vi "uPolicy_TopicIsRelevant.vi"(8 "error in (no error)":errorcluster, 10 "Observed Topic (Lower Case)":string, 11 "SelectTopics in":refnum<class "SelectTopics.lvclass">) -> (0 "error out":errorcluster, 2 "Relevant?":bool, 3 "SelectTopics out":refnum<class "SelectTopics.lvclass">)   [LabVIEW 2021, in "uFramework_pack_uPolicy.lvlib" / "SelectTopics.lvclass"]
uses:
  SelectTopics.lvclass
  SelectTopics.lvclass/SelectTopics.ctl
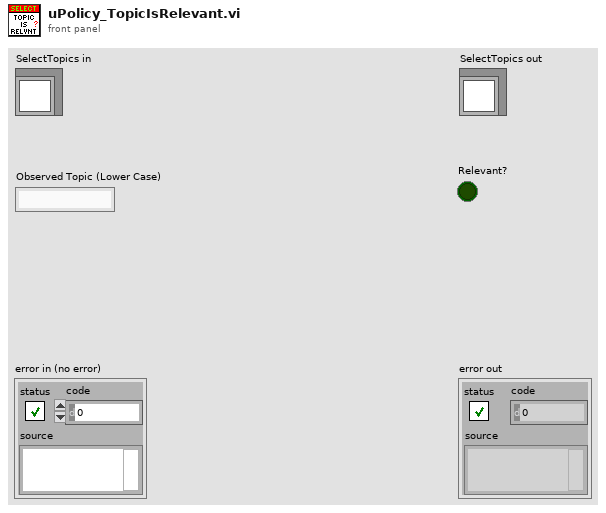
[diagram p1: front panel]
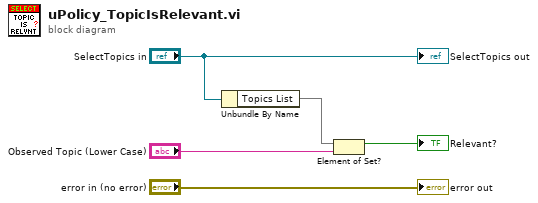
[diagram p0: block diagram]
diagram:
  n1 = Unbundle By Name("SelectTopics in") -> ("Topics List"=w3:set{string})
  n2 = Element of Set?(10:"Observed Topic (Lower Case)", 11:w3) -> (3:→"Relevant?":bool)
  "error out" <- "error in (no error)"
  "SelectTopics out" <- "SelectTopics in"
